vi "Initialize Fluke.vi"(8 "error in (no error)":errorcluster, 11 "Magna Power in":refnum<class "Magna Power.lvclass">) -> (0 "error out":errorcluster, 3 "Magna Power out":refnum<class "Magna Power.lvclass">)   [LabVIEW 2023, in "Magna Power.lvclass"]
uses:
  Magna Power.lvclass
  Magna Power.lvclass/Magna Power.ctl
  Fluke Multimeter/Fluke Multimeter.lvclass
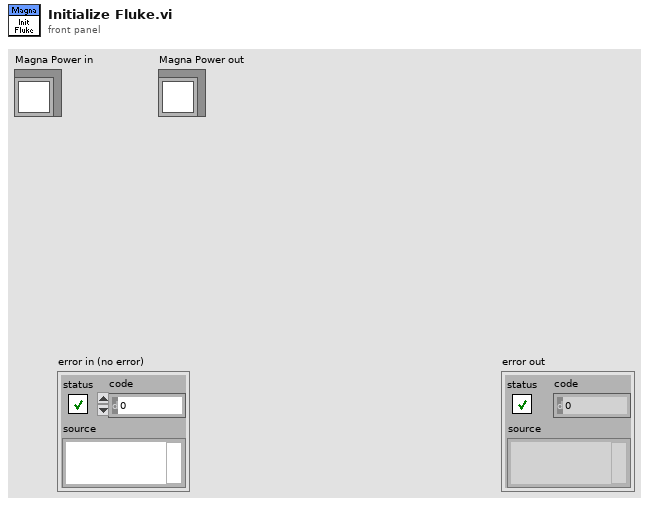
[diagram p1: front panel]
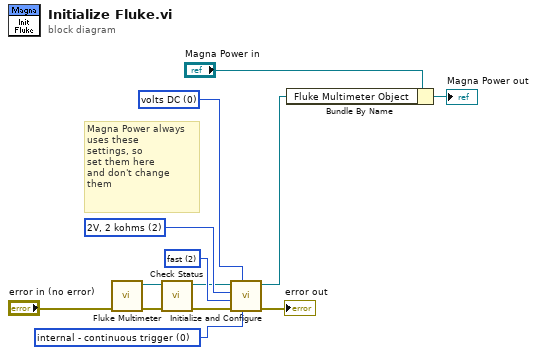
[diagram p0: block diagram]
diagram:
  w13 = u16 0 items=["volts DC", "volts AC", "2-wire k.ohms", "4-wire k.ohms", "mA DC", "mA AC"] ("function (0:volts DC)")
  w12 = u16 2 items=["autorange", "200mV, 200 ohms", "2V, 2 kohms", "20V, 20 kohms", "200V, 200 kohms", "1000Vdc, 700 Vac, 2 Mohms", "20 Mohms", "20 mV, 20 ohms"] ("range (0:auto)")
  w11 = u16 2 items=["slow", "medium", "fast"] ("rate (0:slow)")
  w10 = u16 0 items=["internal - continuous trigger", "external - rear panel trigger with delay", "external - bus trigger with delay", "external - rear panel trigger", "external - bus trigger"] ("trigger mode (0:internal)")
  # "Magna Power always\nuses these\nsettings, so\nset them here\nand don't change\nthem"
  n1 = call "Fluke Multimeter.vi"("error in (no error)"="error in (no error)") -> ("error out"=w8:errorcluster, "Fluke Multimeter out"=w7:refnum<class "Fluke Multimeter.lvclass">)  [unwired: 9 in]
  n2 = call-dynamic "Check Status.vi"("error in (no error)"=w8, "Fluke Multimeter in"=w7) -> ("error out"=w9:errorcluster, "Fluke Multimeter out"=w6:refnum<class "Fluke Multimeter.lvclass">)  [unwired: 6 in, 2 out]
  n3 = call "Initialize and Configure.vi"("trigger mode (0:internal)"=w10, "function (0:volts DC)"=w13, "error in (no error)"=w9, "rate (0:slow)"=w11, "range (0:auto)"=w12, "Fluke Multimeter.lvclass In"=w6) -> ("error out"=→"error out":errorcluster, "Fluke Multimeter.lvclass Out"=w5:refnum<class "Fluke Multimeter.lvclass">)  [unwired: 4 in]
  n4 = Bundle By Name(cluster="Magna Power in", "Fluke Multimeter Object"=w5) -> (→"Magna Power out":refnum<class "Magna Power.lvclass">)
